vi "Inst.Xeryon-Rotator.sendCommand.vi"(8 "error in (no error)":errorcluster, 9 "Value":string, 10 "Command":string, 11 "Inst.Xeryon-Rotator in":refnum<class "Inst.Xeryon-Rotator.lvclass">) -> (0 "error out":errorcluster, 3 "Inst.Xeryon-Rotator out":refnum<class "Inst.Xeryon-Rotator.lvclass">)   [LabVIEW 2019, in "Inst.Xeryon-Rotator.lvclass"]
uses:
  Inst.Xeryon-Rotator.lvclass
  Inst.Xeryon-Rotator.lvclass/Inst.Xeryon-Rotator.ctl
  Controller.LV/Controller.LV.lvclass
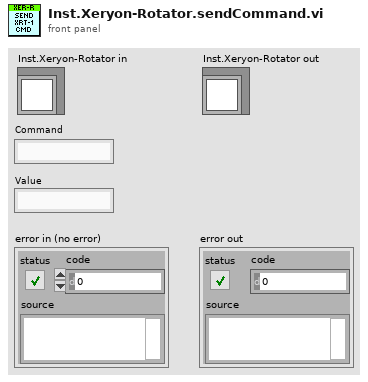
[diagram p1: front panel]
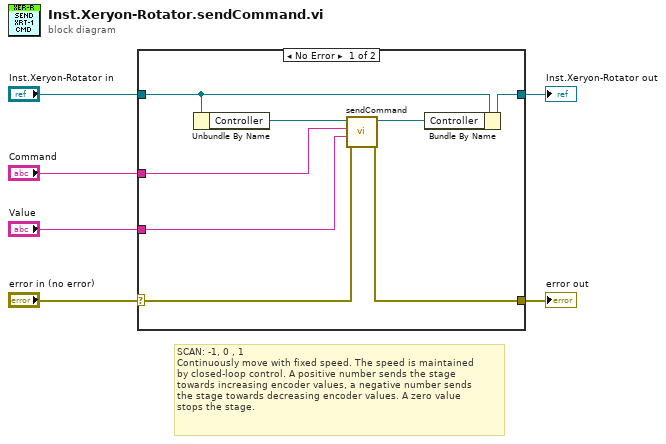
[diagram p0: block diagram]
diagram:
  # "SCAN: -1, 0 , 1\nContinuously move with fixed speed. The speed is maintained\nby closed-loop control. A positive number sends the stage\ntowards increasing encoder values, a negative number sends\nthe stage towards decreasing encoder values. A zero value\nstops the stage."
  n1 = case shown="No Error" "error in (no error)" {
    selector: "error in (no error)" -> [w11 w16]
    tunnel: "Inst.Xeryon-Rotator in" -> [w13 w15]
    tunnel: [w10 w16] -> w4
    tunnel: [w9 w15] -> w3
    tunnel: "Value" -> [w8 _]
    tunnel: "Command" -> [w7 _]
    frame No Error {
      n2 = Unbundle By Name(w13) -> ("Controller"=w14:refnum<class "Controller.LV.lvclass">)
      n3 = call-dynamic "sendCommand.vi"("error in (no error)"=w11, "Value"=w8, "Command"=w7, "Controller in"=w14) -> ("error out"=w10:errorcluster, "Controller out"=w12:refnum<class "Controller.LV.lvclass">)  [unwired: 6 in]
      n4 = Bundle By Name(cluster=w13, "Controller"=w12) -> (w9:refnum<class "Inst.Xeryon-Rotator.lvclass">)
    }
    frame Error {
    }
  }
  "Inst.Xeryon-Rotator out" <- w3
  "error out" <- w4
